vi "Date.vi"(3 "DATE":timestamp format="%<%d/%m/%Y>T", 11 "Message":string) -> ()   [LabVIEW 2015]
panel:
  in  "OK Button":bool
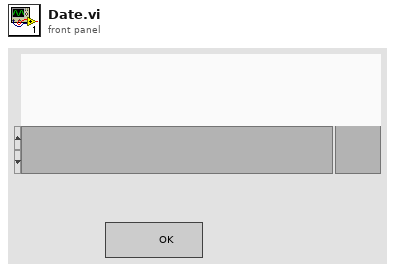
[diagram p1: front panel]
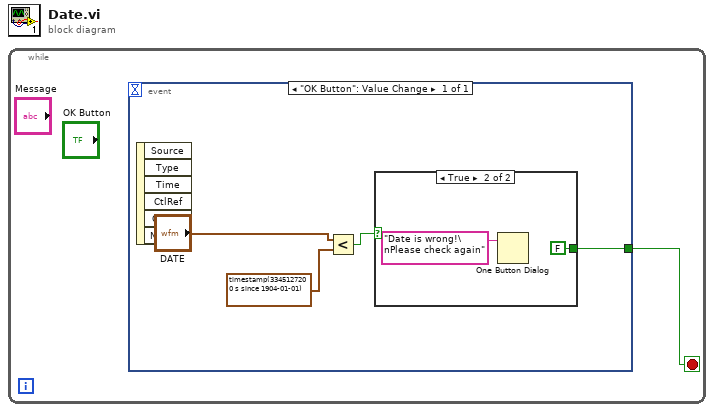
[diagram p0: block diagram]
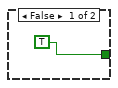
[diagram p2: hidden frame]
diagram:
  n1 = while {
    stop <- w1 stop-if-true
    n2 = event shown="[0] \"OK Button\": Value Change" {
      selector: _ -> [_]
      dyn-events: _ -> [_]
      timeout: _ -> [_]
      tunnel: [w2] -> w1
      event "OK Button": Value Change {
        n3 = event-data() -> ()  [unwired: 1 in, 6 out]
        n4 = Less?(x="DATE", y=timestamp(3345127200 s since 1904-01-01)) -> (x < y?=w3:bool)
        n5 = case shown="True" w3 {
          tunnel: [TRUE FALSE] -> w2
          frame False {
          }
          frame True {
            n6 = One Button Dialog(message="Date is wrong!\nPlease check again") -> ()  [unwired: 1 in, 1 out]
          }
        }
      }
    }
  }
